vi "emi_Get DateTime In Seconds offs.vi"() -> (8 "Time":timestamp)   [LabVIEW 2010]
doc: "Same As Get Date/Time In Seconds. But has an Error IO\n\nOn Error In: No change\n\nSubroutine Reentrant"
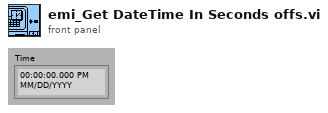
[diagram p1: front panel]
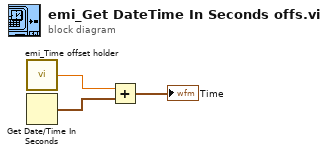
[diagram p0: block diagram]
diagram:
  n1 = call "emi_Time offset holder.vi"() -> ("Offset out"=w1:dbl)  [unwired: 15 in]
  n2 = Get Date/Time In Seconds() -> (seconds since 1Jan1904=w3:timestamp)
  n3 = Add(x=w1, y=w3) -> (x+y=→"Time":timestamp)
